vi "initCAN_backup.vi"(2 "BaudRate":u32=500000, 3 "SlotNum":u32, 4 "CAN":cluster{"Interface":refnum<k21>[], "Slot":u32[]}) -> ()   [LabVIEW 2021]
uses:
  <vilib>/xnet/xnet.llb/XNET Create Session (Frame Input Stream).vi
  <vilib>/xnet/xnet.llb/XNET Create Session (Frame Output Stream).vi
  <resource>/objmgr/xnet.rc
panel:
  out "CANout":T1
  out "error out":errorcluster
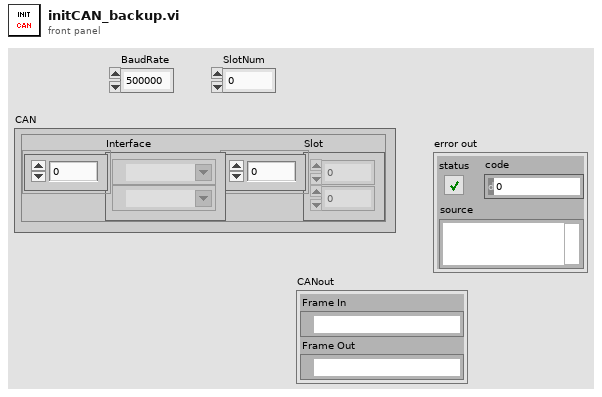
[diagram p1: front panel]
types:
  T1 = cluster{"Frame In":refnum<k21>, "Frame Out":refnum<k21>}
  T2 = cluster{"session out":refnum<k21>, "session out":refnum<k21>}
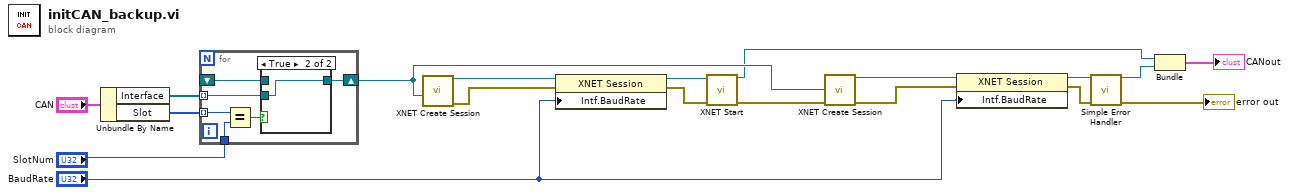
[diagram p0: block diagram]
diagram:
  n1 = Unbundle By Name("CAN") -> ("Interface"=w7:refnum<k21>[], "Slot"=w8:u32[])
  n2 = for {
    tunnel: w8 -> [w24] mode=indexing
    tunnel: w7 -> [w22] mode=indexing
    shift-right: [w21] -> w5
    shift-left: _ -> [w20]
    tunnel: "SlotNum" -> [w19]
    n3 = Equal?(x=w24, y=w19) -> (x = y?=w23:bool)
    n4 = case shown="True" w23 {
      tunnel: w22 -> [_ w26]
      tunnel: [w25 w26] -> w21
      tunnel: w20 -> [w25 _]
      frame False {
      }
      frame True {
      }
    }
  }
  n5 = call-poly <vilib>:"XNET Create Session.vi"("interface"=w5) -> ("session out"=w16:refnum<k21>, "error out"=w17:errorcluster)  [unwired: 2 in, 11 out]
  n6 = property class="XNET Session"(reference=w16, error in=w17, "Intf.BaudRate"="BaudRate") -> (reference out=w14:refnum<k21>, error out=w13:errorcluster)
  n7 = call <vilib>:"XNET Start.vi"("session in"=w14, "error in (no error)"=w13) -> ("session out"=w3:refnum<k21>, "error out"=w12:errorcluster)  [unwired: 12 out]
  n8 = call-poly <vilib>:"XNET Create Session.vi"("interface"=w5, "error in (no error)"=w12) -> ("session out"=w18:refnum<k21>, "error out"=w11:errorcluster)  [unwired: 1 in, 11 out]
  n9 = property class="XNET Session"(reference=w18, error in=w11, "Intf.BaudRate"="BaudRate") -> (reference out=w1:refnum<k21>, error out=w15:errorcluster)
  n10 = call <vilib>:"Simple Error Handler.vi"("error in (no error)"=w15) -> ("error out"=→"error out":errorcluster)  [unwired: 4 in, 4 out]
  n11 = Bundle("session out"=w3, "session out"=w1) -> (→"CANout":T2)  [unwired: 1 in]
